vi "AssertSubpanelExecStateNotBad_Tests.vi"(11 "error in":errorcluster) -> (15 "error out":errorcluster)   [LabVIEW 2016, in "DronaTest.lvlib"]
uses:
  DronaTest.lvlib
  APIs/Stimulus/ControlValue/ValueSignalByPathString.vi
  APIs/Assert/AssertControlValue/Controls/Subpanel/AssertSubpanelVIExecNotBad.vi
  <vilib>/addons/_JKI Toolkits/Caraya/classes/Assert/Assert True.vi
  <vilib>/addons/_JKI Toolkits/Caraya/classes/Test/Test.lvclass
  Drona.lvlib
  APIs/Stimulus/ControlValue/ControlValue.lvlib
  <vilib>/addons/_JKI Toolkits/Caraya/classes/Assert/Assert.lvclass
  APIs/Assert/AssertControlValue/Controls/Subpanel/AssertSubpanel.lvlib
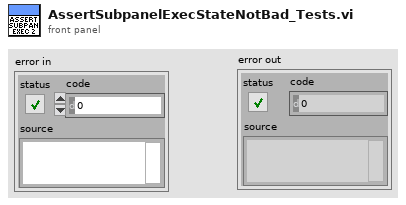
[diagram p1: front panel]
types:
  T1 = enum32{"Bad", "Idle", "Run top level", "Running"}[]
  T2 = enum32{"Bad", "Idle", "Run top level", "Running"}
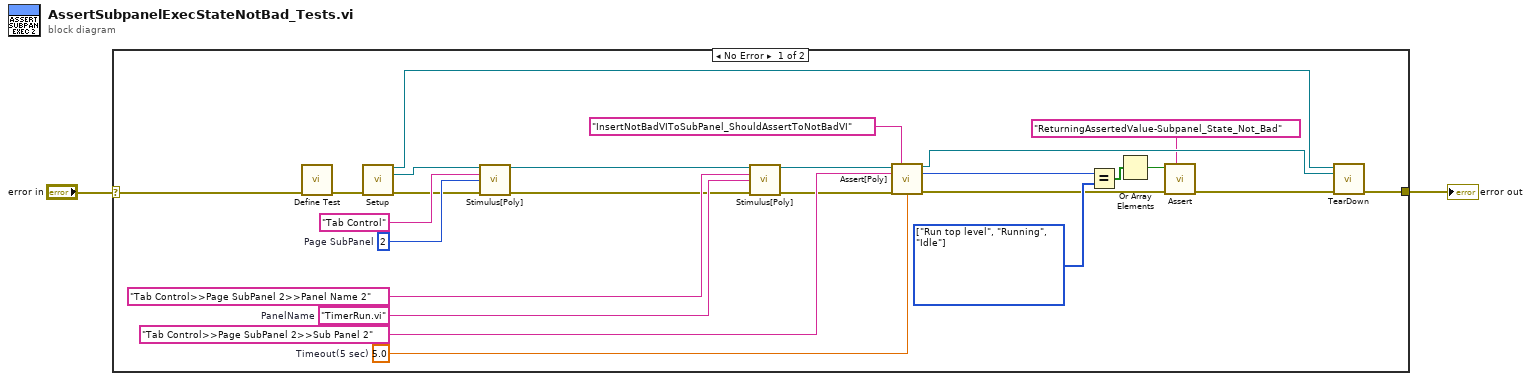
[diagram p0: block diagram]
diagram:
  n1 = case shown="No Error" "error in" {
    selector: "error in" -> [w26 w28]
    tunnel: [w13 w28] -> w1
    frame No Error {
      w7 = T1 [enum."Run top level", enum."Running", enum."Idle"] items=["Bad", "Idle", "Run top level", "Running"] ("Execution:State")
      w17 = 2  # Page SubPanel
      w22 = "TimerRun.vi"  # PanelName
      w23 = 5.0  # Timeout(5 sec)
      n2 = call <vilib>:"Define Test.vi"("error in (no error)"=w26) -> ("error out"=w19:errorcluster)  [unwired: 9 in, 1 out]
      n3 = call "Setup.vi"("error in"=w19) -> ("Application Ref"=w11:refnum<vi>, "VI out"=w10:refnum<vi>, "error out"=w14:errorcluster)  [unwired: 12 in]
      n4 = call-poly "Stimulus[Poly].vi"("VI Reference In"=w10, "Control Path"="Tab Control", "Value (Signaling)"=w17, "error in"=w14) -> ("VI Reference Out"=w20:refnum<vi>, "error out"=w16:errorcluster)  [unwired: 10 in]
      n5 = call-poly "Stimulus[Poly].vi"("VI Reference In"=w20, "Control Path"="Tab Control>>Page SubPanel 2>>Panel Name 2", "Value (Signaling)"=w22, "error in"=w16) -> ("VI Reference Out"=w15:refnum<vi>, "error out"=w21:errorcluster)  [unwired: 10 in]
      n6 = call-poly "Assert[Poly].vi"("VI Reference In"=w15, "Test Label"="InsertNotBadVIToSubPanel_ShouldAssertToNotBadVI" ("Label"), "Control Path"="Tab Control>>Page SubPanel 2>>Sub Panel 2", "Error In"=w21, "Timeout(5 sec)"=w23) -> ("VI Reference Out"=w12:refnum<vi>, "Asserted Value"=w6:T2, "Error Out"=w4:errorcluster)  [unwired: 8 in]
      n7 = Equal?(x=w6, y=w7) -> (x = y?=w5:bool[])
      n8 = Or Array Elements(Boolean array=w5) -> (logical OR=w9:bool)
      n9 = call-poly <vilib>:"Assert.vi"("Label"="ReturningAssertedValue-Subpanel_State_Not_Bad", "error in (no error)"=w4, "True?"=w9) -> ("error out"=w3:errorcluster)  [unwired: 7 in, 1 out]
      n10 = call "TearDown.vi"("Application Ref"=w11, "VI in"=w12, "error in (no error)"=w3) -> ("error out"=w13:errorcluster)  [unwired: 12 in]
    }
    frame Error {
    }
  }
  "error out" <- w1
